vi "Process.vi"(8 "error in":errorcluster, 11 "Instrument.VRM in":refnum<class "Instrument.OxfordVRM.lvclass">) -> (0 "error out":errorcluster, 3 "Instrument.VRM out":refnum<class "Instrument.OxfordVRM.lvclass">)   [LabVIEW 2019, in "Instrument.OxfordVRM.lvclass"]
doc: "---------------------------------------------------------------\nJKI State Machine Objects™\nhttp://jki.net/state-machine-objects/\nCopyright (C) 2005-2015, JKI <info@jki.net>\nALL RIGHTS RESERVED"
uses:
  Instrument.OxfordVRM.lvclass
  <vilib>/JKI/JKI SMO/SMO/SMO.lvclass
  Typedefs/VRM Magnet Axis--Enum.ctl
  <userlib>/LevyLab/Instrument Framework/Instrument Types/Cryostat/Instrument.Cryostat.lvclass
  <userlib>/LevyLab/Instrument Framework/Instrument/Instrument.lvclass
  <userlib>/LevyLab/Debug/Debug.lvlib
  Typedefs/Instrument.VRM.SetTarget--cluster.ctl
  <userlib>/LevyLab/Instrument Framework/Instrument Types/Cryostat/Typedefs/Magnet Mode--Enum.ctl
  <userlib>/LevyLab/Instrument Framework/Instrument Types/Cryostat/Typedefs/Magnet Axis--Enum.ctl
  <userlib>/LevyLab/Instrument Framework/Instrument Types/Cryostat/Typedefs/setMagnet--cluster.ctl
  <userlib>/LevyLab/Instrument Framework/Instrument Types/Cryostat/Typedefs/setMagnetVector--cluster.ctl
  C:/Program Files/National Instruments/LabVIEW 2019/user.lib/LevyLab/Instrument Framework/Instrument Types/Cryostat/Instrument.Cryostat.lvclass
  C:/Program Files/National Instruments/LabVIEW 2019/user.lib/LevyLab/Instrument Framework/Instrument/Instrument.lvclass
  C:/Program Files/National Instruments/LabVIEW 2019/vi.lib/JKI/JKI SMO/SMO/SMO.lvclass
  Typedefs/Instrument.VRM.protectedCommands-enum.ctl
  <userlib>/LevyLab/Instrument Framework/Instrument/API/Instrument.sendMessageToProcess (variant).vi
  <userlib>/LevyLab/Instrument Framework/Instrument/Typedefs/Client Type--Enum.ctl
panel:
  out "Timer":string
  out "State History":string
  out "timer":u32
  # "VRM"
  # "VRM"
  # "For instructions on how to use the JKI State Machine Objects, examples and video tutorials, visit:\nhttp://jki.net/state-machine-objects/\n\nJKI State Machine Objects™\nhttp://jki.net/state-machine-objects/\nCopyright (C) 2005-2015, JKI <info@jki.net>\nALL RIGHTS RESERVED"
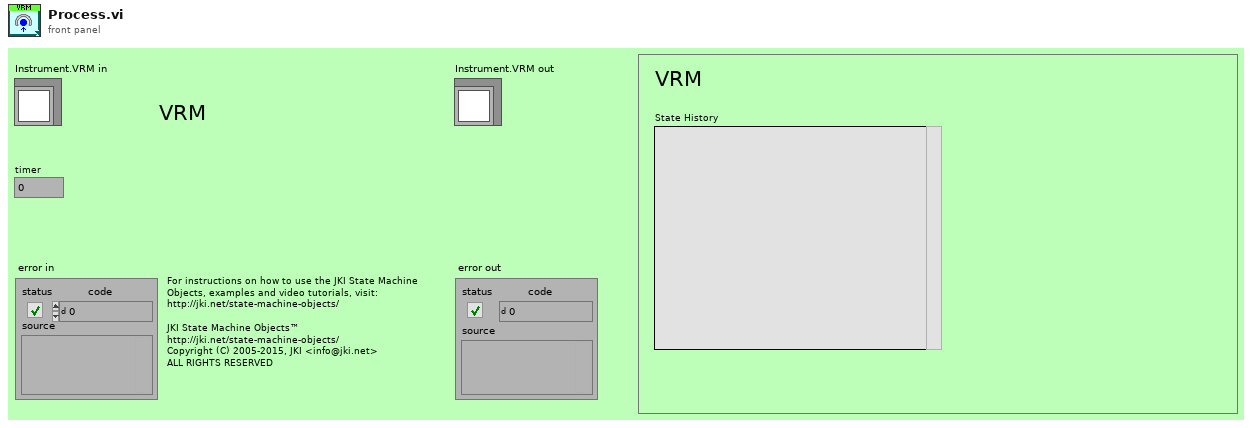
[diagram p1: front panel]
types:
  T1 = typedef "Instrument.OxfordVRM.lvclass/VRM Magnet Axis--Enum.ctl" = enum16{"X", "Y", "Z", "ALL"}
  T2 = typedef "Instrument.OxfordVRM.lvclass/Instrument.VRM.SetTarget--cluster.ctl" = cluster{"field":dbl[], "rate":dbl, "axis":T1}
  T3 = typedef "Instrument.Cryostat.lvclass/setMagnet--cluster.ctl" = cluster{"field":dbl, "rate":dbl, "axis":T4, "mode":T5}
  T4 = typedef "Instrument.Cryostat.lvclass/Magnet Axis--Enum.ctl" = enum16{"X", "Y", "Z"}
  T5 = typedef "Instrument.Cryostat.lvclass/Magnet Mode--Enum.ctl" = enum16{"Persistent", "Driven"}
  T6 = typedef "Instrument.Cryostat.lvclass/setMagnetVector--cluster.ctl" = cluster{"field":dbl[], "rate":dbl}
  T7 = enum32{"invalid app kind", "Development System", "Run Time System", "Student Edition", "Embedded LabVIEW", "Evaluation", "Custom"}
  T8 = enum32{"Invalid", "Standard", "Closed", "Hidden", "Minimized", "Maximized"}
  T9 = typedef "Instrument.OxfordVRM.lvclass/Instrument.VRM.protectedCommands-enum.ctl" = enum16{"Hold", "RampToSet", "RampToZero", "Clamp", "SetTarget", "GetStatus", "GetTarget", "GetField", "setSequenceStatus"}
  T10 = typedef "Instrument.lvlib/Instrument.lvclass/Client Type--Enum.ctl" = enum16{"Remote", "Local"}
  T11 = cluster{"Core":cluster{"Current VI Reference":refnum<vi>, "Close Panel on Exit?":bool, "Last Error":cluster{"error":errorcluster, "previous state":string, "remaining states":string}, "Shutdown?":bool}, "SMO":refnum<class "Instrument.OxfordVRM.lvclass">, "Field (T)":dbl[], "Field Rate (T/min)":dbl, "Axis":T1, "Running Step":i32, "sequence":string[]}
  T12 = cluster{"Current VI Reference":refnum<vi>, "Close Panel on Exit?":bool, "Last Error":cluster{"error":errorcluster, "previous state":string, "remaining states":string}, "Shutdown?":bool}
  T13 = typedef "Instrument.OxfordVRM.lvclass/getAll.ctl" = cluster{"Field":dbl[], "Target Field":dbl[], "Target Field Rate":dbl[], "PSU Current":dbl[], "PSU Voltage":dbl[], "Status":string[]}
  T14 = typedef "Debug.lvlib/Attribute.Debug.lvclass/DebugBehavior.ctl" = enum16{"Normal", "Debug"}
  T15 = typedef "SMO.lvclass/Protected Events.ctl" = cluster{"StopProcesses":refnum<user-event>, "AbortProcesses":refnum<user-event>, "Config Changed":refnum<user-event>, "Dependency":refnum<user-event>}
  T16 = typedef "Instrument.OxfordVRM.lvclass/PrivateEvents--Cluster.ctl" = cluster{"SendMessageToProcess":refnum<user-event>, "AbortSequence":refnum<user-event>}
  T17 = cluster{"Holding":bool, "Ramp to Setpoint":bool, "Ramp to Zero":bool, "Clamp":bool}
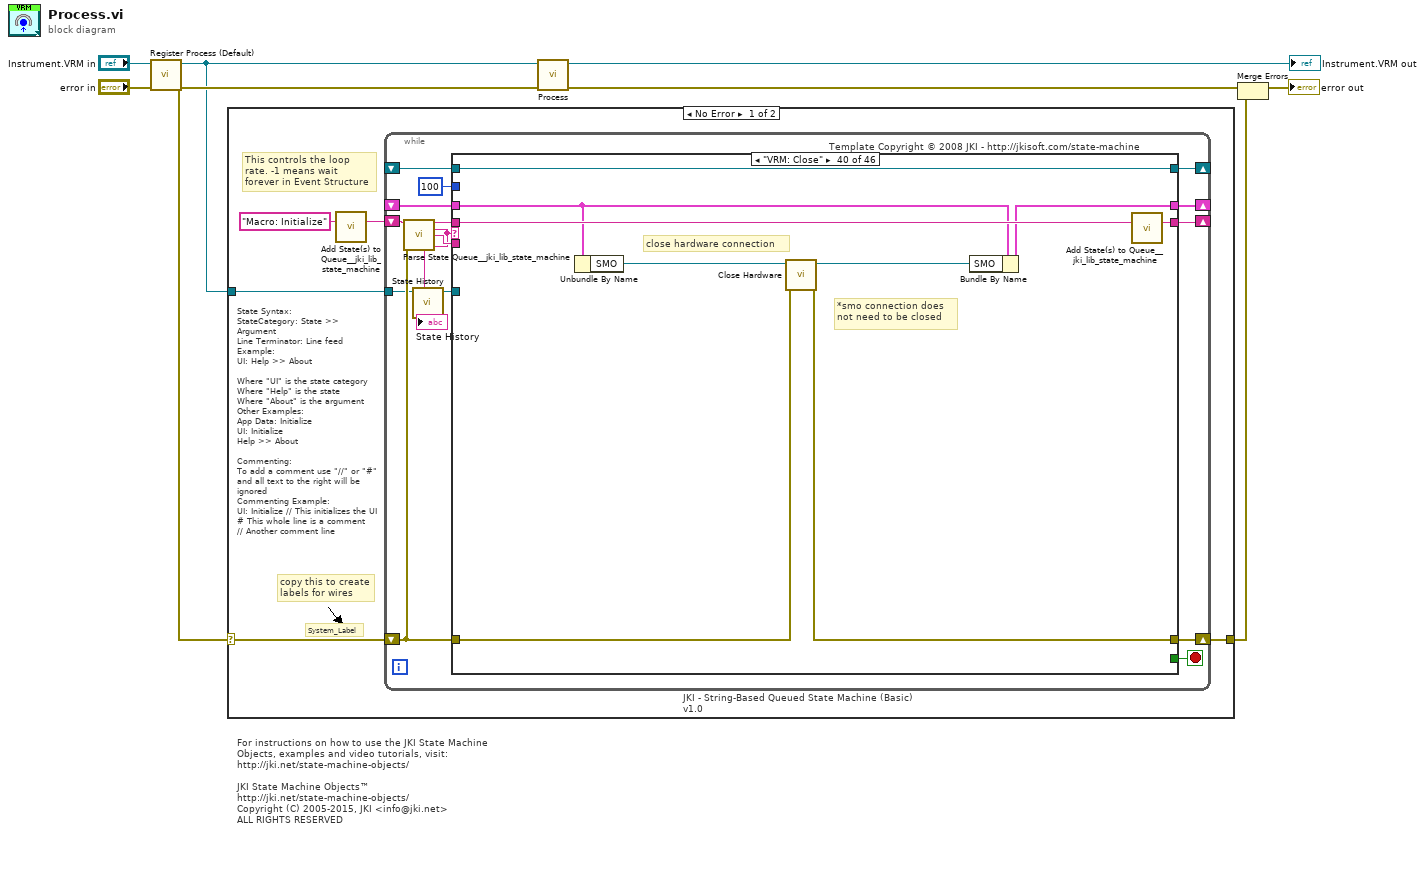
[diagram p0: block diagram]
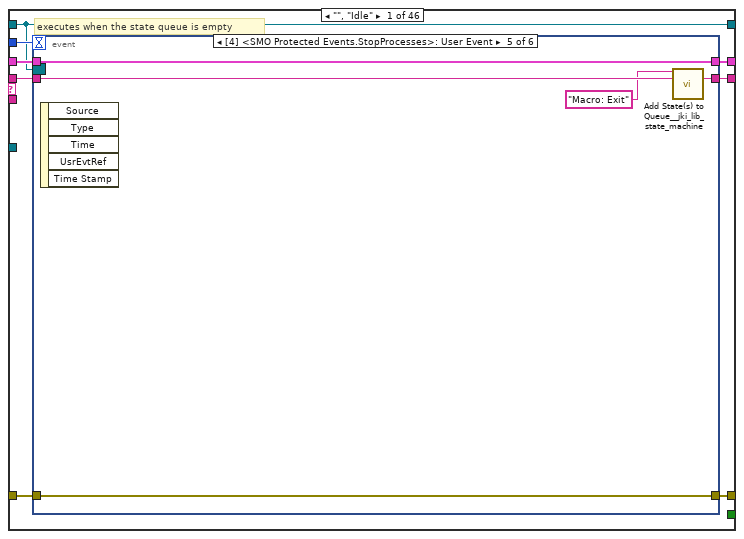
[diagram p2: hidden frame]
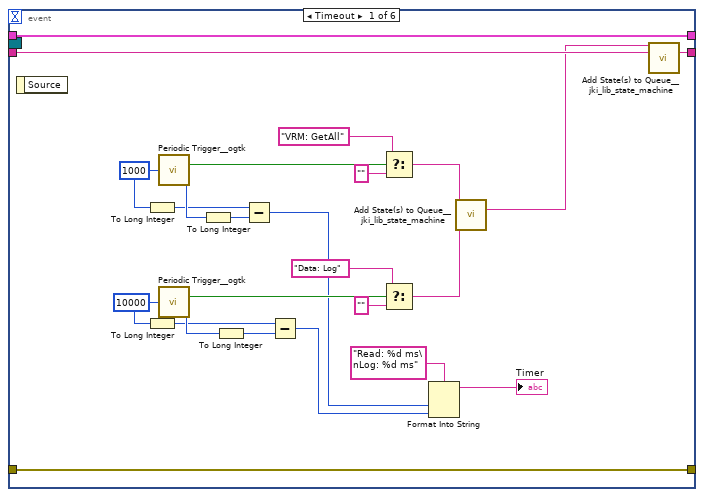
[diagram p3: hidden frame]
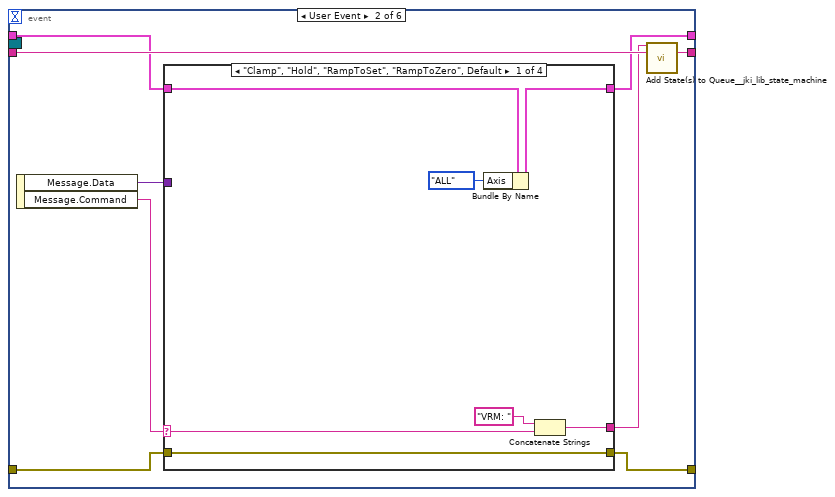
[diagram p4: hidden frame]
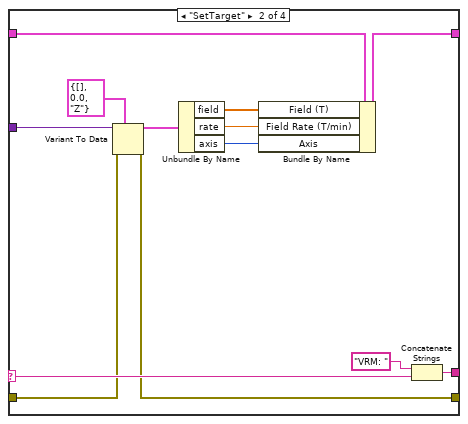
[diagram p5: hidden frame]
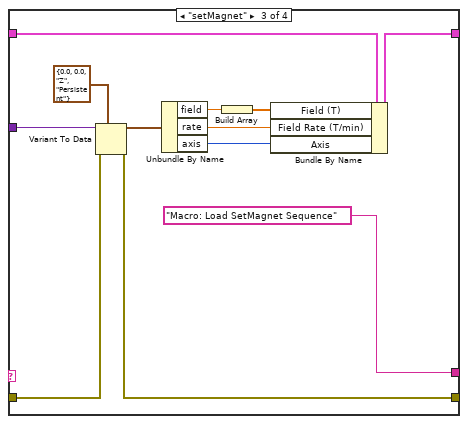
[diagram p6: hidden frame]
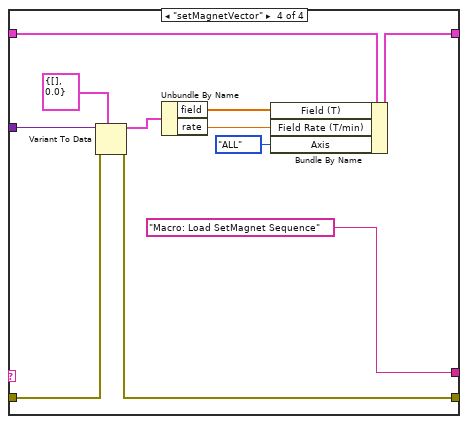
[diagram p7: hidden frame]
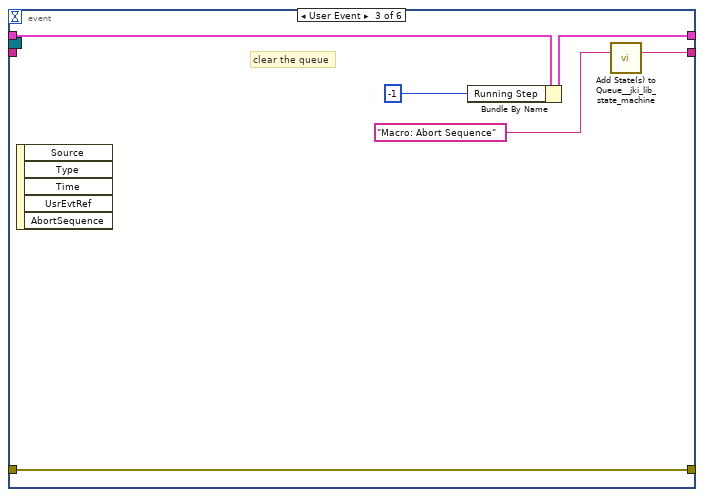
[diagram p8: hidden frame]
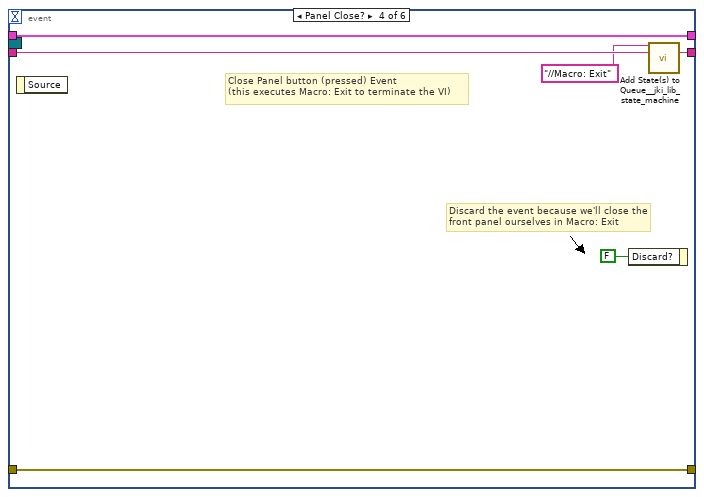
[diagram p9: hidden frame]
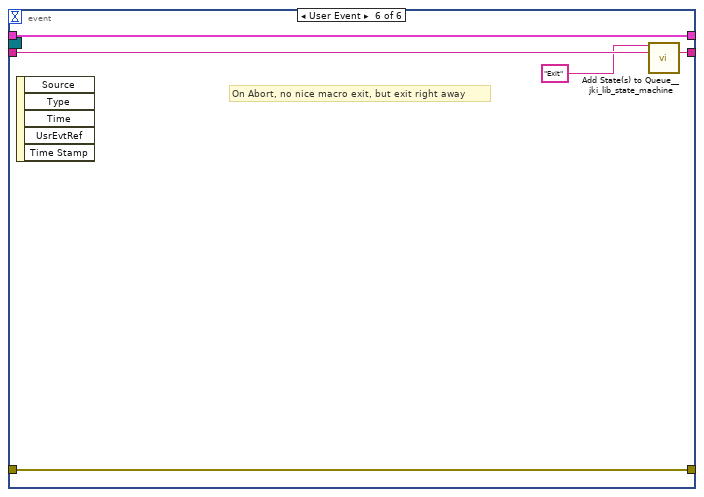
[diagram p10: hidden frame]
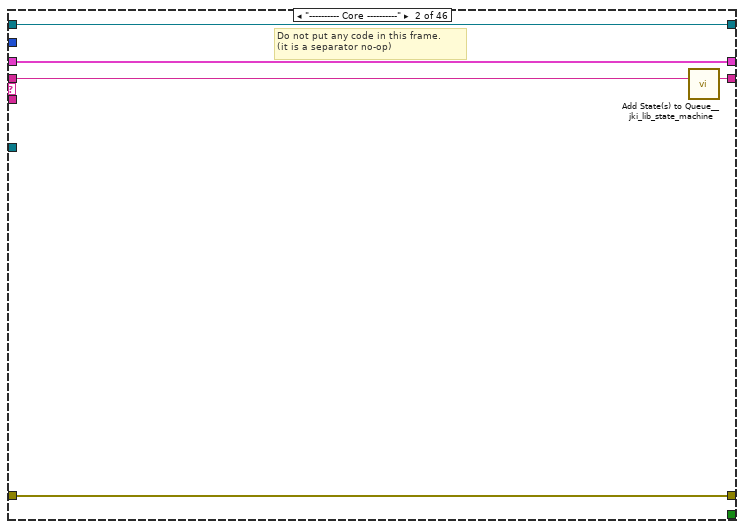
[diagram p11: hidden frame]
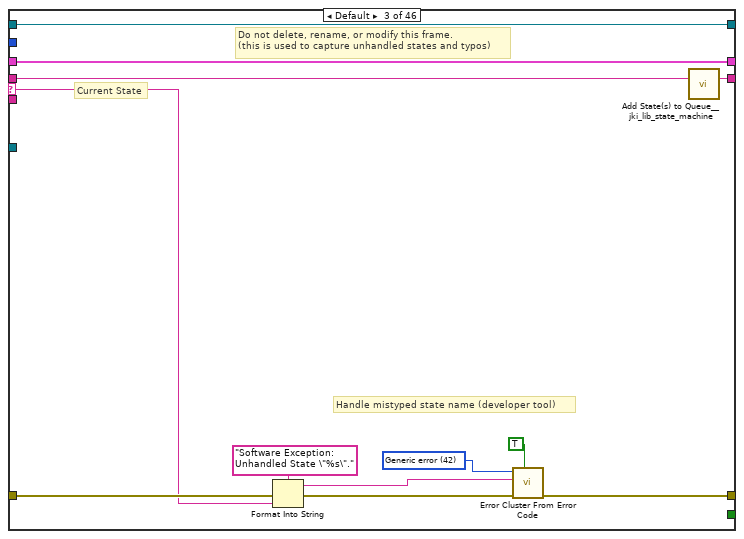
[diagram p12: hidden frame]
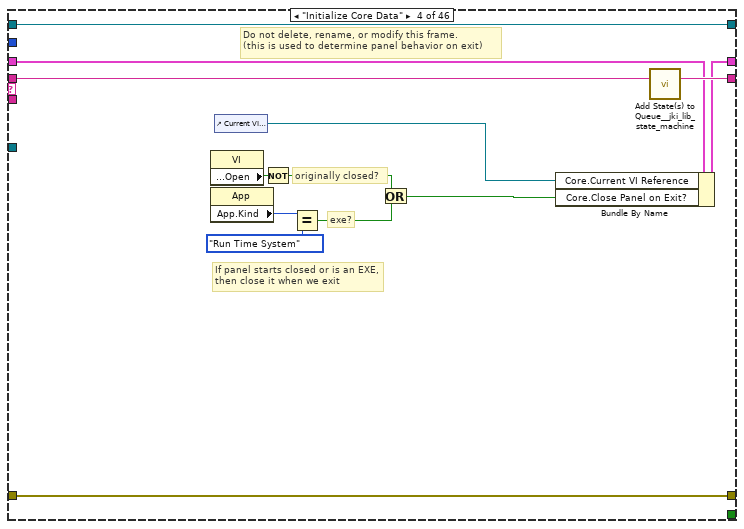
[diagram p13: hidden frame]
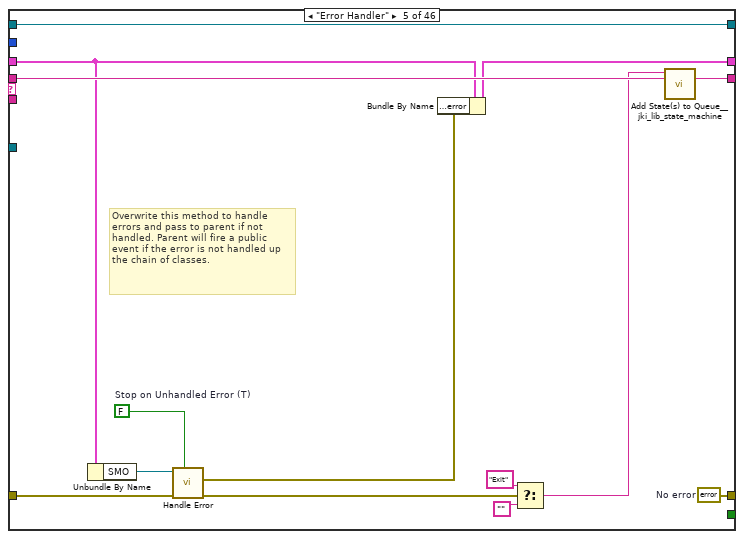
[diagram p14: hidden frame]
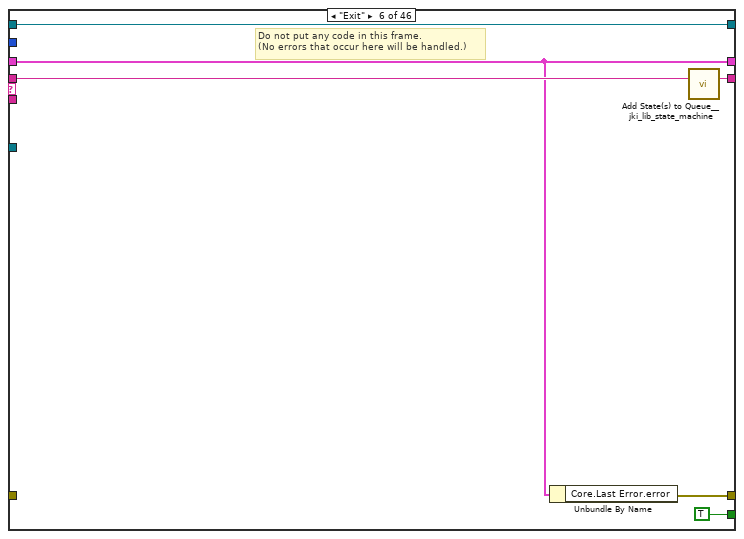
[diagram p15: hidden frame]
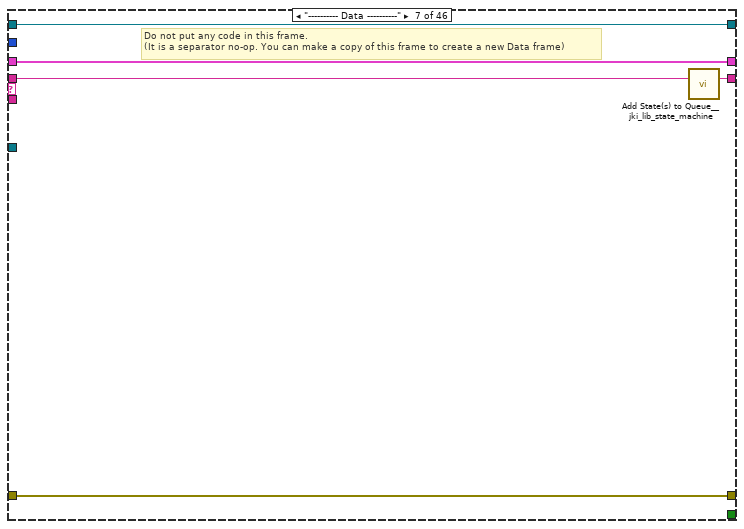
[diagram p16: hidden frame]
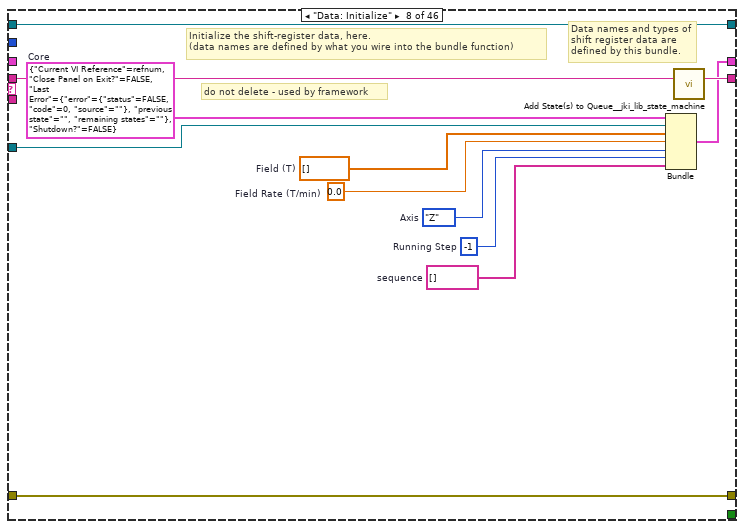
[diagram p17: hidden frame]
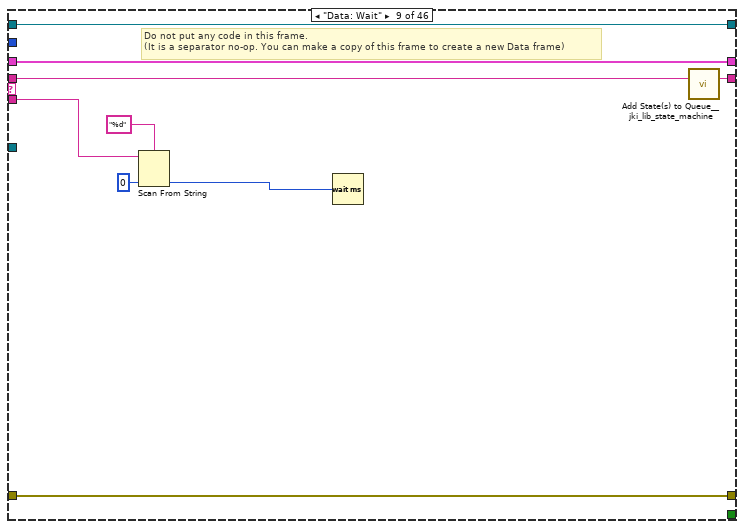
[diagram p18: hidden frame]
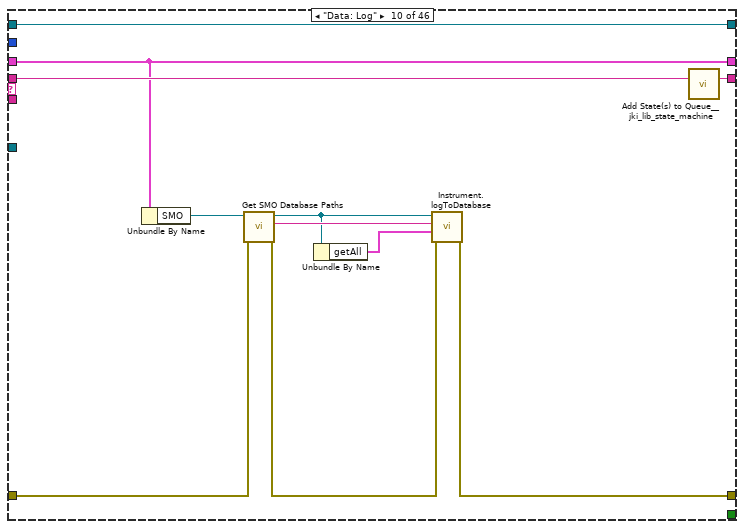
[diagram p19: hidden frame]
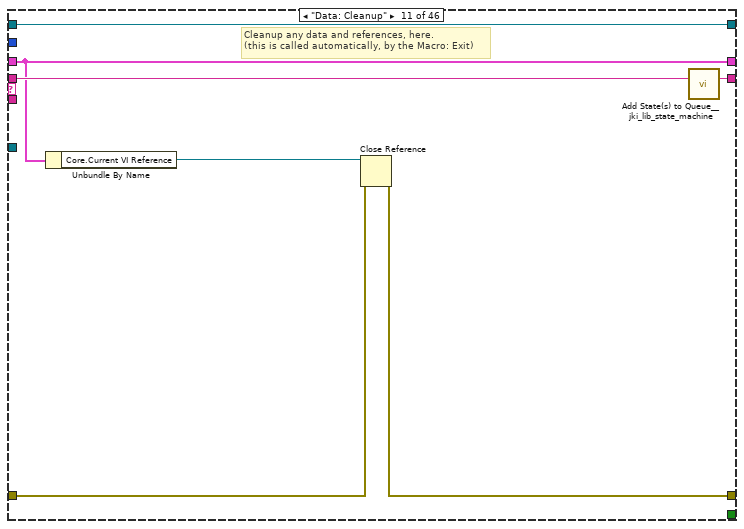
[diagram p20: hidden frame]
diagram:
  # "For instructions on how to use the JKI State Machine Objects, examples and video tutorials, visit:\nhttp://jki.net/state-machine-objects/\n\nJKI State Machine Objects™\nhttp://jki.net/state-machine-objects/\nCopyright (C) 2005-2015, JKI <info@jki.net>\nALL RIGHTS RESERVED"
  n1 = call <vilib>:"Register Process (Default).vi"("error in (no error)"="error in", "SMO"="Instrument.VRM in") -> ("error out"=w5:errorcluster, "SelfRef"=w4:refnum<class "Instrument.OxfordVRM.lvclass">)  [unwired: 8 in]
  n2 = case shown="No Error" w5 {
    selector: w5 -> [w10 w760]
    tunnel: w4 -> [w11 _]
    tunnel: [w9 w760] -> w1
    frame No Error {
      # "State Syntax:\nStateCategory: State >> Argument\nLine Terminator: Line feed\nExample:\nUI: Help >> About\n\nWhere \"UI\" is the state category\nWhere \"Help\" is the state\nWhere \"About\" is the argument\nOther Examples:\nApp Data: Initialize\nUI: Initialize\nHelp >> About\n\nCommenting:\nTo add a comment use \"//\" or \"#\" and all text to the right will be ignored\nCommenting Example:\nUI: Initialize // This initializes the UI\n# This whole line is a comment\n// Another comment line"
      # "copy this to create labels for wires"
      # "This controls the loop rate. -1 means wait forever in Event Structure"
      # "System_Label"
      n3 = call <vilib>:"Add State(s) to Queue__jki_lib_state_machine.vi"("State(s) in (\"\")"="Macro: Initialize") -> ("States Out"=w13:string)  [unwired: 14 in]
      n4 = while "JKI - String-Based Queued State Machine (Basic) v1.0" {
        shift-right: [w23] -> _
        shift-left: _ -> [w22]
        shift-right: [w26] -> w9
        shift-left: w10 -> [w20]
        shift-right: [w25] -> _
        shift-left: w13 -> [w27]
        tunnel: w11 -> [w15]
        shift-right: [w19] -> _
        shift-left: _ -> [w18]
        stop <- w24 stop-if-true
        # "Template Copyright © 2008 JKI - http://jkisoft.com/state-machine"
        n5 = call <vilib>:"Parse State Queue__jki_lib_state_machine.vi"("State Queue"=w27, "Error In (no error)"=w20) -> ("Remaining States"=w29:string, "Current State"=w17:string, "Arguments"=w28:string)  [unwired: 11 in]
        n6 = call <userlib>:"State History.vi"("Current State"=w17, "SMO"=w15) -> ("SMO"=w16:refnum<class "Instrument.OxfordVRM.lvclass">, "History"=→"State History":string)  [unwired: 8 in]
        n7 = case shown="\"VRM: Close\"" w17 {
          selector: w17 -> [_ _ w143 _ _ _ _ _ _ _ _ _ _ _ _ _ _ _ _ _ _ _ _ _ _ _ _ _ _ _ w495 _ w540 w562 w584 w607 w631 _ _ _ _ w688 w703 w718 w734 w751]
          tunnel: w29 -> [w37 w141 w147 w166 w180 w186 w191 w203 w212 w223 w230 w235 w242 w251 w258 w274 w306 w315 w330 w351 w368 _ _ w427 w438 w443 w456 w462 w471 w478 w507 w528 w550 w572 w594 w617 w640 w649 w661 w670 w682 w697 w712 w727 w742 w759]
          tunnel: w28 -> [_ _ _ _ _ _ _ _ w204 _ _ _ _ w244 w252 w268 _ _ _ _ _ _ _ _ _ _ _ _ _ _ w496 w518 _ _ _ _ _ _ _ _ _ _ _ _ _ _]
          tunnel: w22 -> [w35 w138 w145 w157 w174 w182 w188 _ w209 w220 w225 w232 w240 w248 w256 w270 w303 w312 w318 w336 w356 w378 w416 w424 w428 w440 w454 w460 w463 w474 w481 w523 w543 w565 w587 w614 w637 w643 w655 w662 w677 w694 w709 w724 w739 w756]
          tunnel: [w34 w139 w149 w163 w175 w181 w189 w192 w210 w213 w226 w233 w237 w249 w253 w271 w304 w307 w317 w349 w366 w375 w415 w425 w430 w441 w449 w458 w468 w475 w485 w516 w532 w554 w576 w599 w630 w646 w651 w665 w671 w691 w706 w721 w730 w746] -> w26
          tunnel: w20 -> [w33 w139 w148 w163 w176 _ w189 w192 w210 w214 w227 w233 w236 w249 w254 w272 w304 w307 w316 w349 w366 w376 w415 w425 w431 w441 w450 w458 w468 w475 w484 w524 w531 w553 w575 w601 w625 w646 w657 w664 w676 w685 w700 w716 w731 w747]
          tunnel: [w36 w140 w146 w165 w179 w185 w190 w202 w211 w222 w229 w234 w241 w250 w257 w273 w305 w314 w329 w350 w367 w384 w422 w426 w437 w442 w455 w461 w470 w477 w506 w527 w549 w571 w593 w616 w639 w648 w660 w669 w681 w696 w711 w726 w741 w758] -> w25
          tunnel: [_ _ _ _ _ TRUE _ _ _ _ _ _ _ _ _ _ _ _ _ _ _ _ _ _ _ _ _ _ _ _ _ _ _ _ _ _ _ _ _ _ _ _ _ _ _ _] -> w24
          tunnel: [w32 w138 w145 w164 w173 w182 w188 w201 w209 w220 w225 w232 w240 w248 w256 w270 w303 w312 w319 w337 w364 w379 w417 w424 w428 w440 w454 w460 w465 w473 w479 w522 w542 w564 w586 w613 w636 w642 w656 w663 w678 w693 w708 w723 w738 w755] -> w23
          tunnel: 100 ("Timeout") -> [w31 _ _ _ _ _ _ _ _ _ _ _ _ _ _ _ _ _ _ _ _ _ _ _ _ _ _ _ _ _ _ _ _ _ _ _ _ _ _ _ _ _ _ _ _ _]
          tunnel: w16 -> [_ _ _ _ _ _ _ w193 _ _ _ _ _ _ _ _ _ _ _ _ _ _ _ _ _ _ _ _ _ _ _ _ _ _ _ _ _ _ _ _ _ _ _ _ _ _]
          tunnel: [w30 w137 w142 w154 w178 w183 w187 w200 w208 w221 w224 w231 w239 w243 w255 w267 w302 w313 w328 w343 w365 w383 w421 w423 w436 w439 w453 w459 w469 w476 w505 w526 w548 w570 w592 w615 w638 w647 w659 w668 w680 w695 w710 w725 w740 w757] -> w19
          tunnel: w18 -> [w30 w137 w142 w154 w178 w183 w187 w200 w208 w221 w224 w231 w239 w243 w255 w267 w302 w313 w328 w343 w365 w383 w421 w423 w436 w439 _ w459 w469 w476 w505 w526 w548 w570 w592 w615 w638 w647 w659 w668 w680 w695 w710 w725 w740 w757]
          frame "", "Idle" {
            # "executes when the state queue is empty"
            n8 = event shown="[4] <SMO Protected Events.StopProcesses>: User Event" {
              selector: w30 -> [_ _ _ _ _ _]
              dyn-events: _ -> [_ _ _ _ _ _]
              timeout: w31 -> [_ _ _ _ _ _]
              tunnel: w37 -> [w62 w70 _ w126 w131 w136]
              tunnel: [w61 w71 w119 w125 w130 w135] -> w36
              tunnel: w35 -> [w59 w69 w117 w123 w128 w133]
              tunnel: [w60 w65 w120 w124 w129 w134] -> w34
              tunnel: w33 -> [w60 w64 w120 w124 w129 w134]
              tunnel: [w59 w68 w116 w123 w128 w133] -> w32
              event Timeout {
                w47 = u32 10000 ("time (ms)")
                w49 = u32 1000 ("time (ms)")
                n9 = event-data() -> ()  [unwired: 1 in, 1 out]
                n10 = To Long Integer(number=w49) -> (32bit integer=w40:i32)
                n11 = To Long Integer(number=w47) -> (32bit integer=w41:i32)
                n12 = call <userlib>:"Periodic Trigger__ogtk.vi"("time (ms)"=w49) -> ("Triggered"=w58:bool, "timer value"=w48:u32)  [unwired: 12 in, 1 out]
                n13 = call <userlib>:"Periodic Trigger__ogtk.vi"("time (ms)"=w47) -> ("Triggered"=w53:bool, "timer value"=w46:u32)  [unwired: 12 in, 1 out]
                n14 = To Long Integer(number=w48) -> (32bit integer=w39:i32)
                n15 = To Long Integer(number=w46) -> (32bit integer=w38:i32)
                n16 = Subtract(x=w40, y=w39) -> (x-y=w45:i32)
                n17 = Subtract(x=w41, y=w38) -> (x-y=w44:i32)
                n18 = Select(t="VRM: GetAll" ("State(s) in Front (\"\")"), s=w58, f="") -> (s? t:f=w51:string)
                n19 = Select(t="Data: Log" ("State(s) in Front (\"\")"), s=w53, f="") -> (s? t:f=w52:string)
                n20 = Format Into String(format string="Read: %d ms\nLog: %d ms", w45, w44) -> (resulting string=→"Timer":string)  [unwired: 2 in, 1 out]
                n21 = call <vilib>:"Add State(s) to Queue__jki_lib_state_machine.vi"("State(s) in Front (\"\")"=w51, "State(s) at Back (\"\")"=w52) -> ("States Out"=w50:string)  [unwired: 13 in]
                n22 = call <vilib>:"Add State(s) to Queue__jki_lib_state_machine.vi"("State(s) in Front (\"\")"=w50, "State(s) in (\"\")"=w62) -> ("States Out"=w61:string)  [unwired: 13 in]
              }
              event User Event {
                n23 = event-data() -> ("Message.Data"=w66:variant, "Message.Command"=w63:string)  [unwired: 1 in]
                n24 = case shown="\"Clamp\", \"Hold\", \"RampToSet\", \"RampToZero\", Default" w63 {
                  selector: w63 -> [w77 w90 _ _]
                  tunnel: w69 -> [w72 w88 w103 w114]
                  tunnel: [w73 w87 w102 w113] -> w68
                  tunnel: [w78 w91 "Macro: Load SetMagnet Sequence" ("State(s) at Back (\"\")") "Macro: Load SetMagnet Sequence" ("State(s) at Back (\"\")")] -> w67
                  tunnel: w66 -> [_ w85 w99 w110]
                  tunnel: w64 -> [w75 w81 w97 w109]
                  tunnel: [w75 w80 w96 w108] -> w65
                  frame "Clamp", "Hold", "RampToSet", "RampToZero", Default {
                    n25 = Bundle By Name(cluster=w72, "Axis"=VRM_Magnet_Axis--Enum."ALL") -> (w73:T11)
                    n26 = Concatenate Strings("VRM: " ("State"), w77) -> (w78:string)
                  }
                  frame "SetTarget" {
                    n27 = Variant To Data(error in=w81, type=T2 {"field"=[], "rate"=0.0, "axis"=enum."Z"} ("setTarget"), Variant=w85) -> (data=w79:T2, error out=w80:errorcluster)
                    n28 = Unbundle By Name(w79) -> ("field"=w84:dbl[], "rate"=w83:dbl, "axis"=w82:T1)
                    n29 = Bundle By Name(cluster=w88, "Field (T)"=w84, "Field Rate (T/min)"=w83, "Axis"=w82) -> (w87:T11)
                    n30 = Concatenate Strings("VRM: " ("State"), w90) -> (w91:string)
                  }
                  frame "setMagnet" {
                    n31 = Variant To Data(error in=w97, type=T3 {"field"=0.0, "rate"=0.0, "axis"=enum."Z", "mode"=enum."Persistent"} ("setMagnet"), Variant=w99) -> (data=w100:T3, error out=w96:errorcluster)
                    n32 = Unbundle By Name(w100) -> ("field"=w93:dbl, "rate"=w94:dbl, "axis"=w95:T4)
                    n33 = Build Array(w93) -> (w92:dbl[])
                    n34 = Bundle By Name(cluster=w103, "Field (T)"=w92, "Field Rate (T/min)"=w94, "Axis"=w95) -> (w102:T11)
                  }
                  frame "setMagnetVector" {
                    n35 = Variant To Data(error in=w109, type=T6 {"field"=[], "rate"=0.0} ("setMagnet"), Variant=w110) -> (data=w111:T6, error out=w108:errorcluster)
                    n36 = Unbundle By Name(w111) -> ("field"=w105:dbl[], "rate"=w107:dbl)
                    n37 = Bundle By Name(cluster=w114, "Field (T)"=w105, "Field Rate (T/min)"=w107, "Axis"=VRM_Magnet_Axis--Enum."ALL") -> (w113:T11)
                  }
                }
                n38 = call <vilib>:"Add State(s) to Queue__jki_lib_state_machine.vi"("State(s) in Front (\"\")"=w67, "State(s) in (\"\")"=w70) -> ("States Out"=w71:string)  [unwired: 13 in]
              }
              event User Event {
                # "clear the queue"
                n39 = event-data() -> ()  [unwired: 1 in, 5 out]
                n40 = Bundle By Name(cluster=w117, "Running Step"=-1) -> (w116:T11)
                n41 = call <vilib>:"Add State(s) to Queue__jki_lib_state_machine.vi"("State(s) in (\"\")"="Macro: Abort Sequence" ("State(s) at Back (\"\")")) -> ("States Out"=w119:string)  [unwired: 14 in]
              }
              event Panel Close? {
                # "Discard the event because we'll close the front panel ourselves in Macro: Exit"
                # "Close Panel button (pressed) Event\n(this executes Macro: Exit to terminate the VI)"
                n42 = event-data() -> ()  [unwired: 1 in, 1 out]
                n43 = event-data("Discard?"=FALSE) -> ()  [unwired: 1 in, 1 out]
                n44 = call <vilib>:"Add State(s) to Queue__jki_lib_state_machine.vi"("State(s) in Front (\"\")"="//Macro: Exit", "State(s) in (\"\")"=w126) -> ("States Out"=w125:string)  [unwired: 13 in]
              }
              event User Event {
                n45 = event-data() -> ()  [unwired: 1 in, 5 out]
                n46 = call <vilib>:"Add State(s) to Queue__jki_lib_state_machine.vi"("State(s) in Front (\"\")"="Macro: Exit", "State(s) in (\"\")"=w131) -> ("States Out"=w130:string)  [unwired: 13 in]
              }
              event User Event {
                # "On Abort, no nice macro exit, but exit right away"
                n47 = event-data() -> ()  [unwired: 1 in, 5 out]
                n48 = call <vilib>:"Add State(s) to Queue__jki_lib_state_machine.vi"("State(s) in Front (\"\")"="Exit", "State(s) in (\"\")"=w136) -> ("States Out"=w135:string)  [unwired: 13 in]
              }
            }
          }
          frame "---------- Core ----------" {
            # "Do not put any code in this frame.\n(it is a separator no-op)"
            n49 = call <vilib>:"Add State(s) to Queue__jki_lib_state_machine.vi"("State(s) in (\"\")"=w141) -> ("States Out"=w140:string)  [unwired: 14 in]
          }
          frame Default {
            w152 = 42 items=["No error", "Argument error", "Memory is full", "Out of zone", "End of file", "File already open", "Generic file I/O error", "File not found", "File permission error", "Disk is full", "Duplicate path", "Too many files open", "System feature not enabled", "Resource file not found", "Cannot add resource", "Resource not found", "Image not found", "Image memory error", "Pen does not exist", "Config type invalid", "Config token not found", "Config parse error", "Config memory error", "Bad external code format", "Bad external code offset", "External code not present", "Null window", "Destroy window error", "Null menu", "Print aborted", "Bad print record", "Print driver error", "Windows error during printing", "Memory error during printing", "Print dialog error", "Generic print error", "Invalid device refnum", "Device not found", "Device parameter error", "Device unit error", "Cannot open device", "Device call aborted", "Generic error", "Cancelled by user", "Object ID too low", "Object ID too high", "Object not in heap", "Unknown heap", "Unknown object (invalid DefProc)", "Unknown object (DefProc not in table)", "Message out of range", "Invalid (null) method", "Unknown message", "Manager call not supported", "Bad address", "Network operation in progress", "Network operation timed out", "Connection is busy", "Network attribute not supported", "Network error", "Address in use", "System out of memory", "Connection aborted", "Connection refused", "Not connected", "Already connected", "Connection closed", "Initialization error (interapplication manager)", "Bad occurrence", "Wait on unbound occurrence handler", "Occurrence queue overflow", "Datalog type conflict", "Unused", "Unrecognized type (interapplication manager)", "Memory corrupt", "Failed to make temporary DLL", "Old CIN version", "Drag socket not found", "Failed to load drop-object", "Failed to register OLE object", "Failed to release OLE object", "Format specifier type mismatch", "Unknown format specifier", "Too few format specifiers", "Too many format specifiers", "Scan failed", "Newer CIN version", "Error converting to variant", "Runtime menu error", "Password tampered", "Variant attribute not found", "Incompatible variant data type", "Event data is not available", "Event Store is not present", "Occurrence is not found", "Event Queue is not created", "Event info is not available", "Refnum passed is NULL", "Error retrieving Class GUID", "Error retrieving CoClass GUID", "Error retrieving TypeLib GUID.", "Bad built application magic bytes.", "Specific driver is different from the specific driver associated with the Logical Name.", "There is no session opened to the class driver.", "Max Error", "MAX - Error with config objects", "MAX - Error loading configuration", "MAX - Group not supported"]
            # "Current State"
            # "Do not delete, rename, or modify this frame.\n(this is used to capture unhandled states and typos)"
            # "Handle mistyped state name (developer tool)"
            n50 = Format Into String(format string="Software Exception: Unhandled State \"%s\"." ("message"), error in=w148, w143) -> (resulting string=w151:string, error out=w150:errorcluster)  [unwired: 1 in]
            n51 = call <vilib>:"Error Cluster From Error Code.vi"("show call chain? (False)"=TRUE, "error in (no error)"=w150, "error message (\"\")"=w151, "error code (0)"=w152) -> ("error out"=w149:errorcluster)  [unwired: 5 in]
            n52 = call <vilib>:"Add State(s) to Queue__jki_lib_state_machine.vi"("State(s) in (\"\")"=w147) -> ("States Out"=w146:string)  [unwired: 14 in]
          }
          frame "Initialize Core Data" {
            # "Do not delete, rename, or modify this frame.\n(this is used to determine panel behavior on exit)"
            # "originally closed?"
            # "exe?"
            # "If panel starts closed or is an EXE, then close it when we exit"
            n53 = property class="VI"() -> ("Front Panel.Open"=w162:bool)  [unwired: 2 in, 2 out]
            n54 = property class="App"() -> ("App.Kind"=w161:T7)  [unwired: 2 in, 2 out]
            n55 = control-ref of="Current VI Reference"() -> (w155:refnum<vi>)
            n56 = Not(x=w162) -> (.not. x?=w159:bool)
            n57 = Equal?(x=w161, y=T7."Run Time System" ("Application:Kind")) -> (x = y?=w158:bool)
            n58 = Or(x=w159, y=w158) -> (x .or. y?=w156:bool)
            n59 = Bundle By Name(cluster=w157, "Core.Current VI Reference"=w155, "Core.Close Panel on Exit?"=w156) -> (w164:T11)
            n60 = call <vilib>:"Add State(s) to Queue__jki_lib_state_machine.vi"("State(s) in (\"\")"=w166) -> ("States Out"=w165:string)  [unwired: 14 in]
          }
          frame "Error Handler" {
            w167 = FALSE  # Stop on Unhandled Error (T)
            w175 = errorcluster {"status"=FALSE, "code"=0, "source"=""}  # No error
            # "Overwrite this method to handle errors and pass to parent if not handled. Parent will fire a public event if the error is not handled up the chain of classes."
            n61 = Unbundle By Name(w174) -> ("SMO"=w177:refnum<class "Instrument.OxfordVRM.lvclass">)
            n62 = call-dynamic "Handle Error.vi"("Stop on Unhandled Error (T)"=w167, "error in"=w176, "SMO"=w177) -> ("handling error"=w168:errorcluster, "Unhandled error"=w171:errorcluster)  [unwired: 6 in, 1 out]
            n63 = Bundle By Name(cluster=w174, "Core.Last Error.error"=w171) -> (w173:T11)
            n64 = Select(t="Exit", s=w168, f="") -> (s? t:f=w172:string)
            n65 = call <vilib>:"Add State(s) to Queue__jki_lib_state_machine.vi"("State(s) in Front (\"\")"=w172, "State(s) in (\"\")"=w180) -> ("States Out"=w179:string)  [unwired: 13 in]
          }
          frame "Exit" {
            # "Do not put any code in this frame.\n(No errors that occur here will be handled.)"
            n66 = Unbundle By Name(w182) -> ("Core.Last Error.error"=w181:errorcluster)
            n67 = call <vilib>:"Add State(s) to Queue__jki_lib_state_machine.vi"("State(s) in (\"\")"=w186) -> ("States Out"=w185:string)  [unwired: 14 in]
          }
          frame "---------- Data ----------" {
            # "Do not put any code in this frame.\n(It is a separator no-op. You can make a copy of this frame to create a new Data frame)"
            n68 = call <vilib>:"Add State(s) to Queue__jki_lib_state_machine.vi"("State(s) in (\"\")"=w191) -> ("States Out"=w190:string)  [unwired: 14 in]
          }
          frame "Data: Initialize" {
            w194 = T12 {"Current VI Reference"=refnum, "Close Panel on Exit?"=FALSE, "Last Error"={"error"={"status"=FALSE, "code"=0, "source"=""}, "previous state"="", "remaining states"=""}, "Shutdown?"=FALSE}  # Core
            w195 = VRM_Magnet_Axis--Enum."Z"  # Axis
            w196 = string[] []  # sequence
            w197 = -1  # Running Step
            w198 = 0.0  # Field Rate (T/min)
            w199 = dbl[] []  # Field (T)
            # "do not delete - used by framework"
            # "Data names and types of shift register data are defined by this bundle."
            # "Initialize the shift-register data, here.\n(data names are defined by what you wire into the bundle function)"
            n69 = Bundle("Core"=w194, "SMO"=w193, "Field (T)"=w199, "Field Rate (T/min)"=w198, "Axis"=w195, "Running Step"=w197, "sequence"=w196) -> (w201:T11)  [unwired: 1 in]
            n70 = call <vilib>:"Add State(s) to Queue__jki_lib_state_machine.vi"("State(s) in (\"\")"=w203) -> ("States Out"=w202:string)  [unwired: 14 in]
          }
          frame "Data: Wait" {
            # "Do not put any code in this frame.\n(It is a separator no-op. You can make a copy of this frame to create a new Data frame)"
            n71 = Scan From String(format string="%d", input string=w204, default 1=u32 0 ("default value 1")) -> (output 1=w205:u32)  [unwired: 2 in, 3 out]
            n72 = Wait (ms)(milliseconds to wait=w205) -> ()  [unwired: 1 out]
            n73 = call <vilib>:"Add State(s) to Queue__jki_lib_state_machine.vi"("State(s) in (\"\")"=w212) -> ("States Out"=w211:string)  [unwired: 14 in]
          }
          frame "Data: Log" {
            n74 = Unbundle By Name(w220) -> ("SMO"=w219:refnum<class "Instrument.OxfordVRM.lvclass">)
            n75 = call-dynamic "Get SMO Database Paths.vi"("error in (no error)"=w214, "Instrument.VRM in"=w219) -> ("error out"=w215:errorcluster, "Paths"=w218:string, "Instrument.VRM out"=w217:refnum<class "Instrument.OxfordVRM.lvclass">)  [unwired: 7 in]
            n76 = Unbundle By Name(w217) -> ("getAll"=w216:T13)
            n77 = call <userlib>:"Instrument.logToDatabase.vi"("error in (no error)"=w215, "Data"=w216, "Paths"=w218, "Instrument"=w217) -> ("error out"=w213:errorcluster)  [unwired: 6 in, 1 out]
            n78 = call <vilib>:"Add State(s) to Queue__jki_lib_state_machine.vi"("State(s) in (\"\")"=w223) -> ("States Out"=w222:string)  [unwired: 14 in]
          }
          frame "Data: Cleanup" {
            # "Cleanup any data and references, here.\n(this is called automatically, by the Macro: Exit)"
            n79 = Unbundle By Name(w225) -> ("Core.Current VI Reference"=w228:refnum<vi>)
            n80 = Close Reference(reference=w228, error in (no error)=w227) -> (error out=w226:errorcluster)
            n81 = call <vilib>:"Add State(s) to Queue__jki_lib_state_machine.vi"("State(s) in (\"\")"=w230) -> ("States Out"=w229:string)  [unwired: 14 in]
          }
          frame "---------- UI ----------" {
            # "Do not put any code in this frame.\n(It is a separator no-op. You can make a copy of this frame to create a new UI frame)"
            n82 = call <vilib>:"Add State(s) to Queue__jki_lib_state_machine.vi"("State(s) in (\"\")"=w235) -> ("States Out"=w234:string)  [unwired: 14 in]
          }
          frame "UI: Initialize" {
            # "Initialize the User Interface, here.\n(this is called automatically, by the Macro: Init)"
            n83 = call <userlib>:"Fit VI window to Largest Dec__ogtk.vi"("error in (no error)"=w236, "border spacing (2 px)"=0) -> ("error out"=w237:errorcluster)  [unwired: 4 in, 1 out]
            n84 = call <vilib>:"Add State(s) to Queue__jki_lib_state_machine.vi"("State(s) in (\"\")"=w242) -> ("States Out"=w241:string)  [unwired: 14 in]
          }
          frame "UI: Wait" {
            n85 = Scan From String(format string="%d", input string=w244, default 1=u32 0 ("default value 1")) -> (output 1=w245:u32)  [unwired: 2 in, 3 out]
            n86 = Wait (ms)(milliseconds to wait=w245) -> ()  [unwired: 1 out]
            n87 = call <vilib>:"Add State(s) to Queue__jki_lib_state_machine.vi"("State(s) in (\"\")"=w251) -> ("States Out"=w250:string)  [unwired: 14 in]
          }
          frame "UI: Cursor Set" {
            # "Argument"
            # "Initialize the User Interface, here.\n(this is called automatically, by the Macro: Init)"
            n88 = disable-structure shown="Default" {
              disable-tunnel: w254 -> [w259 w262]
              disable-tunnel: [w259 w261] -> w253
              disable-tunnel: w252 -> [_ w260]
              frame condition #0 {
              }
              frame condition #1 (active) {
                n89 = case shown="\"Idle\", Default" w260 {
                  tunnel: w262 -> [w264 w266]
                  tunnel: [w263 w265] -> w261
                  frame "Idle", Default {
                    n90 = call <vilib>:"Unset Busy.vi"("error in (no error)"=w264) -> ("error out"=w263:errorcluster)  [unwired: 10 in]
                  }
                  frame "Busy" {
                    n91 = call <vilib>:"Set Busy.vi"("error in (no error)"=w266) -> ("error out"=w265:errorcluster)  [unwired: 9 in, 1 out]
                  }
                }
              }
            }
            n92 = call <vilib>:"Add State(s) to Queue__jki_lib_state_machine.vi"("State(s) in (\"\")"=w258) -> ("States Out"=w257:string)  [unwired: 14 in]
          }
          frame "UI: Front Panel State" {
            # "Argument"
            # "Set Front Panel Open or Closed\n(Usage: \"UI: Front Panel State >> Open|Close\")"
            n93 = Unbundle By Name(w270) -> ("Core.Current VI Reference"=w269:refnum<vi>)
            n94 = disable-structure shown="Default" {
              disable-tunnel: w272 -> [w278 w301]
              disable-tunnel: [w277 w301] -> w271
              disable-tunnel: w269 -> [w276 _]
              disable-tunnel: w268 -> [w275 _]
              frame condition #0 (active) {
                n95 = case shown="\"Close\"" w275 {
                  tunnel: w278 -> [w282 w295]
                  tunnel: [w284 w296] -> w277
                  tunnel: w276 -> [w283 w293]
                  frame "Open", Default {
                    n96 = property class="VI"(reference=w283, error in=w282) -> (reference out=w280:refnum<vi>, error out=w281:errorcluster, "FP.State"=w279:T8)
                    n97 = case shown="\"Closed\"" w279 {
                      tunnel: [w287 w290] -> w284
                      tunnel: w281 -> [w286 w290]
                      tunnel: w280 -> [w285 _]
                      frame "Closed" {
                        n98 = invoke class="VI" method="FP.Open"(reference=w285, error in=w286, "Activate"=TRUE, "State"=T8."Standard") -> (error out=w287:errorcluster)  [unwired: 1 in, 4 out]
                      }
                      frame Default {
                      }
                    }
                  }
                  frame "Close" {
                    n99 = property class="VI"(reference=w293, error in=w295) -> (reference out=w292:refnum<vi>, error out=w294:errorcluster, "FP.State"=w291:T8)
                    n100 = case shown="Default" w291 {
                      tunnel: [w297 w300] -> w296
                      tunnel: w294 -> [w297 w299]
                      tunnel: w292 -> [_ w298]
                      frame "Invalid", "Closed" {
                      }
                      frame Default {
                        n101 = invoke class="VI" method="FP.Close"(reference=w298, error in=w299) -> (error out=w300:errorcluster)  [unwired: 1 in, 2 out]
                      }
                    }
                  }
                }
              }
              frame condition #1 {
              }
            }
            n102 = call <vilib>:"Add State(s) to Queue__jki_lib_state_machine.vi"("State(s) in (\"\")"=w274) -> ("States Out"=w273:string)  [unwired: 14 in]
          }
          frame "---------- Macro ----------" {
            # "Do not put any code in this frame.\n(It is a separator no-op. You can make a copy of this frame to create a new Macro frame)"
            n103 = call <vilib>:"Add State(s) to Queue__jki_lib_state_machine.vi"("State(s) in (\"\")"=w306) -> ("States Out"=w305:string)  [unwired: 14 in]
          }
          frame "Macro: Initialize" {
            # "Initialization Macro\n(This is called once, when the VI starts)"
            n104 = call <vilib>:"Add State(s) to Queue__jki_lib_state_machine.vi"("State(s) in Front (\"\")"="Data: Initialize\nInitialize Core Data\nEvents: Register", "State(s) in (\"\")"="Process: Sync", "State(s) at Back (\"\")"="UI: Initialize\nUI: Front Panel State >> Close\nMacro: Debug\nVRM: Open\nVRM: GetAll") -> ("States Out"=w310:string)  [unwired: 12 in]
            n105 = call <vilib>:"Add State(s) to Queue__jki_lib_state_machine.vi"("State(s) in Front (\"\")"=w310, "State(s) in (\"\")"=w315) -> ("States Out"=w314:string)  [unwired: 13 in]
          }
          frame "Macro: Debug" {
            # "exe?"
            # "If pane is an EXE, then close it when we exit"
            # "Macro: Debug\n(get debug behavior, determine UI and determine shutdown behavior)"
            n106 = Unbundle By Name(w318) -> ("Core.Close Panel on Exit?"=w322:bool, "SMO"=w327:refnum<class "Instrument.OxfordVRM.lvclass">)
            n107 = property class="App"() -> ("App.Kind"=w325:T7)  [unwired: 2 in, 2 out]
            n108 = Equal?(x=w325, y=T7."Run Time System" ("Application:Kind")) -> (x = y?=w321:bool)
            n109 = call <userlib>:"Get Debug Mode.vi"("error in (no error)"=w316, "SMO"=w327) -> ("error out"=w317:errorcluster, "Behavior"=w326:T14)  [unwired: 7 in, 1 out]
            n110 = case shown="\"Normal\", Default" w326 {
              tunnel: [w331 w333] -> w323
              tunnel: w322 -> [w331 _]
              tunnel: w321 -> [_ w335]
              tunnel: [_ "UI: Front Panel State >> Open\nUI: Wait >> 1000"] -> w320
              frame "Normal", Default {
                # "respect core.close"
              }
              frame "Debug" {
                # "keep panel open\nunless exe"
                n111 = Or(x=w335, y=FALSE) -> (x .or. y?=w333:bool)
              }
            }
            n112 = Bundle By Name(cluster=w318, "Core.Close Panel on Exit?"=w323) -> (w319:T11)
            n113 = call <vilib>:"Add State(s) to Queue__jki_lib_state_machine.vi"("State(s) in Front (\"\")"=w320, "State(s) in (\"\")"=w330) -> ("States Out"=w329:string)  [unwired: 13 in]
          }
          frame "Macro: Exit" {
            # "Exit Macro\n(This is called once, when the VI exits)"
            n114 = Unbundle By Name(w336) -> ("Core.Close Panel on Exit?"=w348:bool)
            n115 = Bundle By Name(cluster=w336, "Core.Shutdown?"=TRUE) -> (w337:T11)
            n116 = Select(t="UI: Front Panel State >> Close", s=w348, f="") -> (s? t:f=w345:string)
            n117 = call <vilib>:"Add State(s) to Queue__jki_lib_state_machine.vi"("State(s) in Front (\"\")"="VRM: Close\nData: Cleanup\nEvents: Unregister", "State(s) in (\"\")"="Process: Sync", "State(s) at Back (\"\")"="Exit") -> ("States Out"=w340:string)  [unwired: 12 in]
            n118 = call <vilib>:"Add State(s) to Queue__jki_lib_state_machine.vi"("State(s) in (\"\")"=w345, "State(s) at Back (\"\")"=w340) -> ("States Out"=w344:string)  [unwired: 13 in]
            n119 = call <vilib>:"Add State(s) to Queue__jki_lib_state_machine.vi"("State(s) in Front (\"\")"=w344, "State(s) in (\"\")"=w351) -> ("States Out"=w350:string)  [unwired: 13 in]
          }
          frame "Macro: Run Sequence" {
            # "0,1,2,3,4,"
            # "5"
            # "Do not put any code in this frame.\n(It is a separator no-op. You can make a copy of this frame to create a new Macro frame)"
            n120 = Unbundle By Name(w356) -> ("sequence"=w362:string[], "Running Step"=w354:i32)
            n121 = Index Array(array=w362, index=w354) -> (element=w360:string)
            n122 = Array Size(array=w362) -> (size(s)=w363:i32)
            n123 = Equal?(x=w363, y=w354) -> (x = y?=w355:bool)
            n124 = Select(t=-1 ("Running Step"), s=w355, f=w354) -> (s? t:f=w361:i32)
            n125 = Select(t="Sequence: Update Status >> ...", s=w355, f="Idle\nMacro: Run Sequence" ("State(s) at Back (\"\")")) -> (s? t:f=w357:string)
            n126 = Bundle By Name(cluster=w356, "Running Step"=w361) -> (w364:T11)
            n127 = call <vilib>:"Add State(s) to Queue__jki_lib_state_machine.vi"("State(s) in Front (\"\")"=w360, "State(s) at Back (\"\")"=w357) -> ("States Out"=w359:string)  [unwired: 13 in]
            n128 = call <vilib>:"Add State(s) to Queue__jki_lib_state_machine.vi"("State(s) in Front (\"\")"=w359, "State(s) in (\"\")"=w368) -> ("States Out"=w367:string)  [unwired: 13 in]
          }
          frame "Macro: Load SetMagnet Sequence" {
            # "PUT IN HOLD\nUPDATE TARGET\nRAMP TO TARGET\nCHECK HOLD"
            # "clear the queue"
            n129 = Unbundle By Name(w378) -> ("SMO"=w377:refnum<class "Instrument.OxfordVRM.lvclass">, "Field (T)"=w373:dbl[], "Axis"=w369:T1)
            n130 = call "VRM.Get Field.vi"("Axis"=VRM_Magnet_Axis--Enum."ALL", "error in (no error)"=w376, "Instrument.VRM in"=w377) -> ("error out"=w375:errorcluster, "Field (T)"=w374:dbl[])  [unwired: 6 in, 1 out]
            n131 = case shown="\"ALL\"" w369 {
              tunnel: w374 -> [w387 w391 w397 w403]
              tunnel: w373 -> [w386 w392 w398 w404]
              tunnel: [w385 w393 w399 w405] -> w372
              frame "ALL" {
                n132 = call "Instrument.OxfordVRM.FloatApprox (Array).vi"("y"=w386, "x"=w387) -> ("x ~ y?"=w385:bool)  [unwired: 4 in]
              }
              frame "Z" {
                n133 = Index Array(array=w391, index=2) -> (element=w389:dbl)
                n134 = Index Array(array=w392) -> (element=w390:dbl)  [unwired: 1 in]
                n135 = call "Instrument.OxfordVRM.FloatApprox.vi"("y"=w390, "x"=w389) -> ("x ~ y?"=w393:bool)  [unwired: 4 in]
              }
              frame "X" {
                n136 = Index Array(array=w397, index=0) -> (element=w395:dbl)
                n137 = Index Array(array=w398) -> (element=w396:dbl)  [unwired: 1 in]
                n138 = call "Instrument.OxfordVRM.FloatApprox.vi"("y"=w396, "x"=w395) -> ("x ~ y?"=w399:bool)  [unwired: 4 in]
              }
              frame "Y" {
                n139 = Index Array(array=w403, index=1) -> (element=w401:dbl)
                n140 = Index Array(array=w404) -> (element=w402:dbl)  [unwired: 1 in]
                n141 = call "Instrument.OxfordVRM.FloatApprox.vi"("y"=w402, "x"=w401) -> ("x ~ y?"=w405:bool)  [unwired: 4 in]
              }
            }
            n142 = call <userlib>:"String to 1D Array__ogtk.vi"("delimiter (Tab)"="\n", "string"="VRM: Hold\nSequence: Check Hold\nVRM: SetTarget\nSequence: Check Targets Match\nVRM: RampToSet\nSequence: Check Hold" ("State(s) in Front (\"\")")) -> ("Array of Strings"=w382:string[])  [unwired: 9 in]
            n143 = case shown="False" w372 {
              tunnel: w382 -> [w409 _]
              tunnel: ["Macro: Run Sequence" ("State(s) in Front (\"\")") "" ("State(s) in Front (\"\")")] -> w381
              tunnel: [w407 w411] -> w379
              tunnel: w378 -> [w406 w411]
              frame False {
                n144 = Bundle By Name(cluster=w406, "Running Step"=0 ("sequence"), "sequence"=w409) -> (w407:T11)
              }
              frame True {
              }
            }
            n145 = call <vilib>:"Add State(s) to Queue__jki_lib_state_machine.vi"("State(s) in Front (\"\")"=w381) -> ("States Out"=w384:string)  [unwired: 14 in]
          }
          frame "Macro: Abort Sequence" {
            n146 = call <userlib>:"String to 1D Array__ogtk.vi"("delimiter (Tab)"="\n", "string"="" ("State(s) in Front (\"\")")) -> ("Array of Strings"=w420:string[])  [unwired: 9 in]
            n147 = Bundle By Name(cluster=w416, "Running Step"=0 ("sequence"), "sequence"=w420) -> (w417:T11)
            n148 = call <vilib>:"Add State(s) to Queue__jki_lib_state_machine.vi"("State(s) in Front (\"\")"="Macro: Run Sequence" ("State(s) in Front (\"\")")) -> ("States Out"=w422:string)  [unwired: 14 in]
          }
          frame "---------- Process ----------" {
            # "Template Separator\n(You can make a copy of, or modify, this frame)"
            n149 = call <vilib>:"Add State(s) to Queue__jki_lib_state_machine.vi"("State(s) in (\"\")"=w427) -> ("States Out"=w426:string)  [unwired: 14 in]
          }
          frame "Process: Sync" {
            n150 = Unbundle By Name(w428) -> ("SMO"=w432:refnum<class "Instrument.OxfordVRM.lvclass">)
            n151 = call <vilib>:"WaitOnProcessSync.vi"("error in (no error)"=w431, "SMO"=w432) -> ("error out"=w430:errorcluster, "Don't run?"=w435:bool)  [unwired: 7 in, 1 out]
            n152 = Select(t="Data: Cleanup\nEvents: Unregister\nExit", s=w435, f="") -> (s? t:f=w429:string)
            n153 = call <vilib>:"Add State(s) to Queue__jki_lib_state_machine.vi"("State(s) in Front (\"\")"=w429, "State(s) in (\"\")"=w438) -> ("States Out"=w437:string)  [unwired: 13 in]
          }
          frame "---------- Events ----------" {
            # "Template Separator\n(You can make a copy of, or modify, this frame)"
            n154 = call <vilib>:"Add State(s) to Queue__jki_lib_state_machine.vi"("State(s) in (\"\")"=w443) -> ("States Out"=w442:string)  [unwired: 14 in]
          }
          frame "Events: Register" {
            # "Expand to add\nmore events"
            n155 = Unbundle By Name(w454) -> ("SMO"=w451:refnum<class "Instrument.OxfordVRM.lvclass">)
            n156 = call <vilib>:"GetProtectedEvents.vi"("SMO"=w451) -> ("error out"=w447:errorcluster, "SMO Protected Events"=w452:T15, "SMO out"=w446:refnum<class "Instrument.OxfordVRM.lvclass">)  [unwired: 8 in]
            n157 = call "Instrument.OxfordVRM.GetPrivateEvents.vi"("Instrument.Oxford1820"=w446) -> ("error out"=w445:errorcluster, "Instrument.VRM.Private Events"=w444:T16)  [unwired: 8 in, 1 out]
            n158 = register-events(w452, w444) -> (reference out=w453:refnum<event-registration>, error out=w448:errorcluster)  [unwired: 2 in]
            n159 = Merge Errors(w445, w450, w448, w447) -> (w449:errorcluster)
            n160 = call <vilib>:"Add State(s) to Queue__jki_lib_state_machine.vi"("State(s) in (\"\")"=w456) -> ("States Out"=w455:string)  [unwired: 14 in]
          }
          frame "Events: Unregister" {
            n161 = Unregister For Events(event registration refnum=w459, error in=w458) -> (error out=w457:errorcluster)
            n162 = call <vilib>:"Clear Errors.vi"("error in (no error)"=w457) -> ()  [unwired: 5 in, 2 out]
            n163 = call <vilib>:"Add State(s) to Queue__jki_lib_state_machine.vi"("State(s) in (\"\")"=w462) -> ("States Out"=w461:string)  [unwired: 14 in]
          }
          frame "---------- Sequence ----------" {
            n164 = Unbundle By Name(w463) -> ("Running Step"=w464:i32, "SMO"=w467:refnum<class "Instrument.OxfordVRM.lvclass">)
            n165 = Increment(x=w464) -> (x+1=w466:i32)
            n166 = Bundle By Name(cluster=w463, "Running Step"=w466, "SMO"=w467) -> (w465:T11)
            n167 = call <vilib>:"Add State(s) to Queue__jki_lib_state_machine.vi"("State(s) in (\"\")"=w471) -> ("States Out"=w470:string)  [unwired: 14 in]
          }
          frame "Sequence: Template" {
            n168 = Unbundle By Name(w474) -> ("SMO"=w472:refnum<class "Instrument.OxfordVRM.lvclass">)
            n169 = Bundle By Name(cluster=w474, "SMO"=w472) -> (w473:T11)
            n170 = call <vilib>:"Add State(s) to Queue__jki_lib_state_machine.vi"("State(s) in (\"\")"=w478) -> ("States Out"=w477:string)  [unwired: 14 in]
          }
          frame "Sequence: Wait" {
            # "F = repeat this state. wait\nT = go to next state. don't wait"
            n171 = Unbundle By Name(w481) -> ("Running Step"=w504:i32)
            n172 = Equal?(x=w496, y="RESET") -> (x = y?=w500:bool)
            n173 = case shown="False" w500 {
              tunnel: [w509 u32 10000 ("time (ms)")] -> w499
              tunnel: [w512 w514] -> w486
              tunnel: w484 -> [w511 w514]
              tunnel: w496 -> [w510 _]
              frame False {
                n174 = Scan From String(format string="%d", input string=w510, error in=w511) -> (error out=w512:errorcluster, output 1=w508:i32)  [unwired: 2 in, 2 out]
                n175 = To Unsigned Long Integer(number=w508) -> (unsigned 32bit integer=w509:u32)
              }
              frame True {
              }
            }
            n176 = call <userlib>:"Periodic Trigger__ogtk.vi"("time (ms)"=w499, "reset"=w500) -> ("Triggered"=w501:bool, "timer value"=w498:u32)  [unwired: 11 in, 1 out]
            n177 = Or(x=w501, y=w500) -> (x .or. y?=w483:bool)
            n178 = Increment(x=w504) -> (x+1=w503:i32)
            n179 = Subtract(x=w499, y=w498) -> (x-y=w490:u32)
            "timer" <- w490
            n180 = Select(t=u32 0, s=w483, f=u32 100 ("milliseconds to wait")) -> (s? t:f=w488:u32)
            n181 = Select(t=w503, s=w483, f=w504) -> (s? t:f=w502:i32)
            n182 = call <userlib>:"Wait (ms)__ogtk.vi"("error in (no error)"=w486, "milliseconds to wait"=w488) -> ("error out"=w485:errorcluster)  [unwired: 8 in, 1 out]
            n183 = Bundle By Name(cluster=w481, "Running Step"=w502) -> (w479:T11)
            n184 = Divide(x=w490, y=u32 1000) -> (x/y=w492:dbl)
            n185 = Format Into String(format string="%s >> %d s", w495, w492) -> (resulting string=w493:string)  [unwired: 2 in, 1 out]
            n186 = call <vilib>:"Build State String with Arguments__JKI_lib_State_Machine.vi"("Arguments (\"\")"=w493, "State"="Sequence: Update Status") -> ("State with Arguments"=w480:string)  [unwired: 4 in]
            n187 = call <vilib>:"Add State(s) to Queue__jki_lib_state_machine.vi"("State(s) in Front (\"\")"=w480, "State(s) in (\"\")"=w507) -> ("States Out"=w506:string)  [unwired: 13 in]
          }
          frame "Sequence: Update Status" {
            n188 = Unbundle By Name(w523) -> ("SMO"=w525:refnum<class "Instrument.OxfordVRM.lvclass">)
            n189 = call "Instrument.OxfordVRM.ProcessStatus.vi"("error in (no error)"=w524, "event data"=w518, "Instrument.Oxford1820"=w525) -> ("error out"=w517:errorcluster, "Instrument.Oxford1820 out"=w521:refnum<class "Instrument.OxfordVRM.lvclass">)  [unwired: 7 in]
            n190 = call-poly <userlib>:"Instrument.sendMessageToProcess.vi"("error in (no error)"=w517, "Data"=w518, "Command"=Instrument.VRM.protectedCommands-enum."setSequenceStatus" ("protectedCommands"), "Instrument"=w521) -> ("error out"=w516:errorcluster, "Instrument out"=w520:refnum<class "Instrument.OxfordVRM.lvclass">)  [unwired: 6 in]
            n191 = Bundle By Name(cluster=w523, "SMO"=w520) -> (w522:T11)
            n192 = call <vilib>:"Add State(s) to Queue__jki_lib_state_machine.vi"("State(s) in (\"\")"=w528) -> ("States Out"=w527:string)  [unwired: 14 in]
          }
          frame "Sequence: Check Hold" {
            # "F = repeat this state. wait\nT = go to next state. don't wait"
            n193 = Unbundle By Name(w543) -> ("Running Step"=w545:i32, "SMO"=w539:refnum<class "Instrument.OxfordVRM.lvclass">, "Axis"=w529:T1)
            n194 = call "VRM.Get Status.vi"("Axis"=w529, "error in (no error)"=w531, "Instrument.VRM in"=w539) -> ("error out"=w533:errorcluster, "Status (ALL)"=w547:T17, "Instrument.VRM out"=w530:refnum<class "Instrument.OxfordVRM.lvclass">)  [unwired: 5 in, 1 out]
            n195 = Unbundle By Name(w547) -> ("Holding"=w534:bool)
            n196 = Increment(x=w545) -> (x+1=w546:i32)
            n197 = Select(t=w546, s=w534, f=w545) -> (s? t:f=w544:i32)
            n198 = Select(t=u32 0, s=w534, f=u32 500 ("milliseconds to wait")) -> (s? t:f=w536:u32)
            n199 = Bundle By Name(cluster=w543, "Running Step"=w544, "SMO"=w530) -> (w542:T11)
            n200 = call <userlib>:"Wait (ms)__ogtk.vi"("error in (no error)"=w533, "milliseconds to wait"=w536) -> ("error out"=w532:errorcluster)  [unwired: 8 in, 1 out]
            n201 = call <vilib>:"Build State String with Arguments__JKI_lib_State_Machine.vi"("Arguments (\"\")"=w540, "State"="Sequence: Update Status") -> ("State with Arguments"=w538:string)  [unwired: 4 in]
            n202 = call <vilib>:"Add State(s) to Queue__jki_lib_state_machine.vi"("State(s) in Front (\"\")"=w538, "State(s) in (\"\")"=w550) -> ("States Out"=w549:string)  [unwired: 13 in]
          }
          frame "Sequence: Check RTOS" {
            # "F = repeat this state. wait\nT = go to next state. don't wait"
            n203 = Unbundle By Name(w565) -> ("Running Step"=w567:i32, "SMO"=w561:refnum<class "Instrument.OxfordVRM.lvclass">, "Axis"=w551:T1)
            n204 = call "VRM.Get Status.vi"("Axis"=w551, "error in (no error)"=w553, "Instrument.VRM in"=w561) -> ("error out"=w555:errorcluster, "Status (ALL)"=w569:T17, "Instrument.VRM out"=w552:refnum<class "Instrument.OxfordVRM.lvclass">)  [unwired: 5 in, 1 out]
            n205 = Unbundle By Name(w569) -> ("Ramp to Setpoint"=w556:bool)
            n206 = Increment(x=w567) -> (x+1=w568:i32)
            n207 = Select(t=w568, s=w556, f=w567) -> (s? t:f=w566:i32)
            n208 = Select(t=u32 0, s=w556, f=u32 500 ("milliseconds to wait")) -> (s? t:f=w558:u32)
            n209 = Bundle By Name(cluster=w565, "Running Step"=w566, "SMO"=w552) -> (w564:T11)
            n210 = call <userlib>:"Wait (ms)__ogtk.vi"("error in (no error)"=w555, "milliseconds to wait"=w558) -> ("error out"=w554:errorcluster)  [unwired: 8 in, 1 out]
            n211 = call <vilib>:"Build State String with Arguments__JKI_lib_State_Machine.vi"("Arguments (\"\")"=w562, "State"="Sequence: Update Status") -> ("State with Arguments"=w560:string)  [unwired: 4 in]
            n212 = call <vilib>:"Add State(s) to Queue__jki_lib_state_machine.vi"("State(s) in Front (\"\")"=w560, "State(s) in (\"\")"=w572) -> ("States Out"=w571:string)  [unwired: 13 in]
          }
          frame "Sequence: Check RTOZ" {
            # "F = repeat this state. wait\nT = go to next state. don't wait"
            n213 = Unbundle By Name(w587) -> ("Running Step"=w589:i32, "SMO"=w583:refnum<class "Instrument.OxfordVRM.lvclass">, "Axis"=w573:T1)
            n214 = call "VRM.Get Status.vi"("Axis"=w573, "error in (no error)"=w575, "Instrument.VRM in"=w583) -> ("error out"=w577:errorcluster, "Status (ALL)"=w591:T17, "Instrument.VRM out"=w574:refnum<class "Instrument.OxfordVRM.lvclass">)  [unwired: 5 in, 1 out]
            n215 = Unbundle By Name(w591) -> ("Ramp to Zero"=w578:bool)
            n216 = Increment(x=w589) -> (x+1=w590:i32)
            n217 = Select(t=w590, s=w578, f=w589) -> (s? t:f=w588:i32)
            n218 = Bundle By Name(cluster=w587, "Running Step"=w588, "SMO"=w574) -> (w586:T11)
            n219 = Select(t=u32 0, s=w578, f=u32 500 ("milliseconds to wait")) -> (s? t:f=w580:u32)
            n220 = call <userlib>:"Wait (ms)__ogtk.vi"("error in (no error)"=w577, "milliseconds to wait"=w580) -> ("error out"=w576:errorcluster)  [unwired: 8 in, 1 out]
            n221 = call <vilib>:"Build State String with Arguments__JKI_lib_State_Machine.vi"("Arguments (\"\")"=w584, "State"="Sequence: Update Status") -> ("State with Arguments"=w582:string)  [unwired: 4 in]
            n222 = call <vilib>:"Add State(s) to Queue__jki_lib_state_machine.vi"("State(s) in Front (\"\")"=w582, "State(s) in (\"\")"=w594) -> ("States Out"=w593:string)  [unwired: 13 in]
          }
          frame "Sequence: Check PSU at Zero" {
            # "#todo\nnot needed???"
            # "F = repeat this state. wait\nT = go to next state. don't wait"
            n223 = Unbundle By Name(w614) -> ("Running Step"=w611:i32, "SMO"=w606:refnum<class "Instrument.OxfordVRM.lvclass">, "Axis"=w595:T1)
            n224 = call "VRM.Get Field.vi"("Axis"=w595, "error in (no error)"=w601, "Instrument.VRM in"=w606) -> ("error out"=w600:errorcluster, "Field (T)"=w596:dbl[], "Instrument.VRM out"=w597:refnum<class "Instrument.OxfordVRM.lvclass">)  [unwired: 6 in]
            n225 = call "Instrument.OxfordVRM.FloatApprox (Array).vi"("y"=dbl[] [0.0, 0.0, 0.0], "x"=w596) -> ("x ~ y?"=w602:bool)  [unwired: 4 in]
            n226 = Increment(x=w611) -> (x+1=w612:i32)
            n227 = Select(t=w612, s=w602, f=w611) -> (s? t:f=w610:i32)
            n228 = Bundle By Name(cluster=w614, "Running Step"=w610, "SMO"=w597) -> (w613:T11)
            n229 = Select(t=u32 0, s=w602, f=u32 500 ("milliseconds to wait")) -> (s? t:f=w604:u32)
            n230 = call <userlib>:"Wait (ms)__ogtk.vi"("error in (no error)"=w600, "milliseconds to wait"=w604) -> ("error out"=w599:errorcluster)  [unwired: 8 in, 1 out]
            n231 = call <vilib>:"Build State String with Arguments__JKI_lib_State_Machine.vi"("Arguments (\"\")"=w607, "State"="Sequence: Update Status") -> ("State with Arguments"=w608:string)  [unwired: 4 in]
            n232 = call <vilib>:"Add State(s) to Queue__jki_lib_state_machine.vi"("State(s) in Front (\"\")"=w608, "State(s) in (\"\")"=w617) -> ("States Out"=w616:string)  [unwired: 13 in]
          }
          frame "Sequence: Check Targets Match" {
            # "F = repeat this state. wait\nT = go to next state. don't wait"
            n233 = Unbundle By Name(w637) -> ("Running Step"=w634:i32, "SMO"=w626:refnum<class "Instrument.OxfordVRM.lvclass">, "Field (T)"=w619:dbl[], "Axis"=w618:T1)
            n234 = call "VRM.Get Target.vi"("Axis"=w618, "error in (no error)"=w625, "Instrument.VRM in"=w626) -> ("error out"=w624:errorcluster, "Target Field (T)"=w623:dbl[], "Instrument.VRM out"=w621:refnum<class "Instrument.OxfordVRM.lvclass">)  [unwired: 5 in, 1 out]
            n235 = call "Instrument.OxfordVRM.FloatApprox (Array).vi"("y"=w619, "x"=w623) -> ("x ~ y?"=w620:bool)  [unwired: 4 in]
            n236 = Increment(x=w634) -> (x+1=w635:i32)
            n237 = Select(t=w635, s=w620, f=w634) -> (s? t:f=w633:i32)
            n238 = Select(t=u32 0, s=w620, f=u32 500 ("milliseconds to wait")) -> (s? t:f=w628:u32)
            n239 = call <userlib>:"Wait (ms)__ogtk.vi"("error in (no error)"=w624, "milliseconds to wait"=w628) -> ("error out"=w630:errorcluster)  [unwired: 8 in, 1 out]
            n240 = Bundle By Name(cluster=w637, "Running Step"=w633, "SMO"=w621) -> (w636:T11)
            n241 = call <vilib>:"Build State String with Arguments__JKI_lib_State_Machine.vi"("Arguments (\"\")"=w631, "State"="Sequence: Update Status") -> ("State with Arguments"=w622:string)  [unwired: 4 in]
            n242 = call <vilib>:"Add State(s) to Queue__jki_lib_state_machine.vi"("State(s) in Front (\"\")"=w622, "State(s) in (\"\")"=w640) -> ("States Out"=w639:string)  [unwired: 13 in]
          }
          frame "---------- VRM ----------" {
            n243 = Unbundle By Name(w643) -> ("Running Step"=w641:i32, "SMO"=w645:refnum<class "Instrument.OxfordVRM.lvclass">)
            n244 = Increment(x=w641) -> (x+1=w644:i32)
            n245 = Bundle By Name(cluster=w643, "Running Step"=w644, "SMO"=w645) -> (w642:T11)
            n246 = call <vilib>:"Add State(s) to Queue__jki_lib_state_machine.vi"("State(s) in (\"\")"=w649) -> ("States Out"=w648:string)  [unwired: 14 in]
          }
          frame "VRM: Open" {
            # "connection to parent should \nbe local (ie not through zmq)"
            # "open hardware connection"
            n247 = Unbundle By Name(w655) -> ("SMO"=w658:refnum<class "Instrument.OxfordVRM.lvclass">)
            n248 = call-dynamic "Open Hardware.vi"("error in (no error)"=w657, "Instrument.VRM in"=w658) -> ("error out"=w652:errorcluster, "Instrument.VRM out"=w654:refnum<class "Instrument.OxfordVRM.lvclass">)  [unwired: 8 in]
            n249 = call <userlib>:"Write Client Type.vi"("error in (no error)"=w652, "Client Type [Remote]"=Client_Type--Enum."Local", "Instrument in"=w654) -> ("error out"=w651:errorcluster, "Instrument out"=w653:refnum<class "Instrument.OxfordVRM.lvclass">)  [unwired: 7 in]
            n250 = Bundle By Name(cluster=w655, "SMO"=w653) -> (w656:T11)
            n251 = call <vilib>:"Add State(s) to Queue__jki_lib_state_machine.vi"("State(s) in (\"\")"=w661) -> ("States Out"=w660:string)  [unwired: 14 in]
          }
          frame "VRM: Close" {
            # "*smo connection does\nnot need to be closed"
            # "close hardware connection"
            n252 = Unbundle By Name(w662) -> ("SMO"=w667:refnum<class "Instrument.OxfordVRM.lvclass">)
            n253 = call-dynamic "Close Hardware.vi"("error in (no error)"=w664, "Instrument.VRM in"=w667) -> ("error out"=w665:errorcluster, "Instrument.VRM out"=w666:refnum<class "Instrument.OxfordVRM.lvclass">)  [unwired: 8 in]
            n254 = Bundle By Name(cluster=w662, "SMO"=w666) -> (w663:T11)
            n255 = call <vilib>:"Add State(s) to Queue__jki_lib_state_machine.vi"("State(s) in (\"\")"=w670) -> ("States Out"=w669:string)  [unwired: 14 in]
          }
          frame "VRM: GetAll" {
            n256 = Unbundle By Name(w677) -> ("SMO"=w679:refnum<class "Instrument.OxfordVRM.lvclass">)
            n257 = call "Read IPS All.vi"("error in (no error)"=w676, "Instrument.VRM in"=w679) -> ("error out"=w672:errorcluster, "output cluster"=w674:T13, "Instrument.VRM out"=w675:refnum<class "Instrument.OxfordVRM.lvclass">)  [unwired: 7 in]
            n258 = call <userlib>:"setAllData.vi"("error in (no error)"=w672, "AllData"=w674, "Instrument in"=w675) -> ("error out"=w671:errorcluster, "Instrument out"=w673:refnum<class "Instrument.OxfordVRM.lvclass">)  [unwired: 7 in]
            n259 = Bundle By Name(cluster=w677, "SMO"=w673) -> (w678:T11)
            n260 = call <vilib>:"Add State(s) to Queue__jki_lib_state_machine.vi"("State(s) in (\"\")"=w682) -> ("States Out"=w681:string)  [unwired: 14 in]
          }
          frame "VRM: Hold" {
            n261 = Unbundle By Name(w694) -> ("Running Step"=w687:i32, "SMO"=w683:refnum<class "Instrument.OxfordVRM.lvclass">, "Axis"=w684:T1)
            n262 = Increment(x=w687) -> (x+1=w686:i32)
            n263 = call "VRM.Hold.vi"("Axis"=w684, "error in (no error)"=w685, "Instrument.VRM in"=w683) -> ("error out"=w691:errorcluster, "Instrument.VRM out"=w692:refnum<class "Instrument.OxfordVRM.lvclass">)  [unwired: 6 in, 1 out]
            n264 = Bundle By Name(cluster=w694, "Running Step"=w686, "SMO"=w692) -> (w693:T11)
            n265 = call <vilib>:"Build State String with Arguments__JKI_lib_State_Machine.vi"("Arguments (\"\")"=w688, "State"="Sequence: Update Status") -> ("State with Arguments"=w690:string)  [unwired: 4 in]
            n266 = call <vilib>:"Add State(s) to Queue__jki_lib_state_machine.vi"("State(s) in Front (\"\")"=w690, "State(s) in (\"\")"=w697) -> ("States Out"=w696:string)  [unwired: 13 in]
          }
          frame "VRM: Clamp" {
            n267 = Unbundle By Name(w709) -> ("Running Step"=w702:i32, "SMO"=w699:refnum<class "Instrument.OxfordVRM.lvclass">, "Axis"=w698:T1)
            n268 = Increment(x=w702) -> (x+1=w701:i32)
            n269 = call "VRM.Clamp.vi"("Axis"=w698, "error in (no error)"=w700, "Instrument.VRM in"=w699) -> ("error out"=w706:errorcluster, "Instrument.VRM out"=w707:refnum<class "Instrument.OxfordVRM.lvclass">)  [unwired: 6 in, 1 out]
            n270 = Bundle By Name(cluster=w709, "Running Step"=w701, "SMO"=w707) -> (w708:T11)
            n271 = call <vilib>:"Build State String with Arguments__JKI_lib_State_Machine.vi"("Arguments (\"\")"=w703, "State"="Sequence: Update Status") -> ("State with Arguments"=w705:string)  [unwired: 4 in]
            n272 = call <vilib>:"Add State(s) to Queue__jki_lib_state_machine.vi"("State(s) in Front (\"\")"=w705, "State(s) in (\"\")"=w712) -> ("States Out"=w711:string)  [unwired: 13 in]
          }
          frame "VRM: RampToSet" {
            n273 = Unbundle By Name(w724) -> ("Running Step"=w715:i32, "SMO"=w717:refnum<class "Instrument.OxfordVRM.lvclass">, "Axis"=w713:T1)
            n274 = Increment(x=w715) -> (x+1=w714:i32)
            n275 = call "VRM.Ramp to Set.vi"("Axis"=w713, "error in (no error)"=w716, "Instrument.VRM in"=w717) -> ("error out"=w721:errorcluster, "Instrument.VRM out"=w722:refnum<class "Instrument.OxfordVRM.lvclass">)  [unwired: 6 in, 1 out]
            n276 = Bundle By Name(cluster=w724, "Running Step"=w714, "SMO"=w722) -> (w723:T11)
            n277 = call <vilib>:"Build State String with Arguments__JKI_lib_State_Machine.vi"("Arguments (\"\")"=w718, "State"="Sequence: Update Status") -> ("State with Arguments"=w720:string)  [unwired: 4 in]
            n278 = call <vilib>:"Add State(s) to Queue__jki_lib_state_machine.vi"("State(s) in Front (\"\")"=w720, "State(s) in (\"\")"=w727) -> ("States Out"=w726:string)  [unwired: 13 in]
          }
          frame "VRM: RampToZero" {
            # "#todo: add abort public method"
            # "#todo: make these separate states\n1. check B = Target?\n2. Turn on switch\n3. set PSU to target\n4. check hold OR psu = target\n5. set persist mode"
            n279 = Unbundle By Name(w739) -> ("Running Step"=w737:i32, "SMO"=w732:refnum<class "Instrument.OxfordVRM.lvclass">, "Axis"=w728:T1)
            n280 = call "VRM.Ramp to Zero.vi"("Axis"=w728, "error in (no error)"=w731, "Instrument.VRM in"=w732) -> ("error out"=w730:errorcluster, "Instrument.VRM out"=w729:refnum<class "Instrument.OxfordVRM.lvclass">)  [unwired: 6 in, 1 out]
            n281 = Increment(x=w737) -> (x+1=w736:i32)
            n282 = Bundle By Name(cluster=w739, "Running Step"=w736, "SMO"=w729) -> (w738:T11)
            n283 = call <vilib>:"Build State String with Arguments__JKI_lib_State_Machine.vi"("Arguments (\"\")"=w734, "State"="Sequence: Update Status") -> ("State with Arguments"=w733:string)  [unwired: 4 in]
            n284 = call <vilib>:"Add State(s) to Queue__jki_lib_state_machine.vi"("State(s) in Front (\"\")"=w733, "State(s) in (\"\")"=w742) -> ("States Out"=w741:string)  [unwired: 13 in]
          }
          frame "VRM: SetTarget" {
            n285 = Unbundle By Name(w756) -> ("Running Step"=w754:i32, "SMO"=w750:refnum<class "Instrument.OxfordVRM.lvclass">, "Field (T)"=w749:dbl[], "Field Rate (T/min)"=w748:dbl, "Axis"=w743:T1)
            n286 = Increment(x=w754) -> (x+1=w753:i32)
            n287 = call "VRM.Set Target.vi"("Axis"=w743, "error in (no error)"=w747, "Target Rate Limit (T/min)"=w748, "Target Field (T)"=w749, "Instrument.VRM in"=w750) -> ("error out"=w746:errorcluster, "Instrument.VRM out"=w745:refnum<class "Instrument.OxfordVRM.lvclass">)  [unwired: 5 in]
            n288 = Bundle By Name(cluster=w756, "Running Step"=w753, "SMO"=w745) -> (w755:T11)
            n289 = call <vilib>:"Build State String with Arguments__JKI_lib_State_Machine.vi"("Arguments (\"\")"=w751, "State"="Sequence: Update Status") -> ("State with Arguments"=w752:string)  [unwired: 4 in]
            n290 = call <vilib>:"Add State(s) to Queue__jki_lib_state_machine.vi"("State(s) in Front (\"\")"=w752, "State(s) in (\"\")"=w759) -> ("States Out"=w758:string)  [unwired: 13 in]
          }
        }
      }
    }
    frame Error {
    }
  }
  n291 = call-parent "Process.vi"("error in"=w5, "Instrument"=w4) -> ("error out"=w2:errorcluster, "Instrument out"=→"Instrument.VRM out":refnum<class "Instrument.OxfordVRM.lvclass">)  [unwired: 8 in]
  n292 = Merge Errors(w2, w1) -> (→"error out":errorcluster)
